vi "USB2XXXSPISlaveTest.vi"() -> ()   [LabVIEW 2010]
panel:
  out "Read Data(Hex)":string
  in  "Write Data(Hex)":string="11 22 33 44 55 66 77 88"
  in  "pConfig":T1
  in  "Channel Index":i32(ring) items=["SPI1_CS0", "SPI2_CS0"]
  in  "Device Index":i32(ring) items=["0", "1", "2", "3", "4", "5"]
  in  "Read":bool
  in  "Write":bool
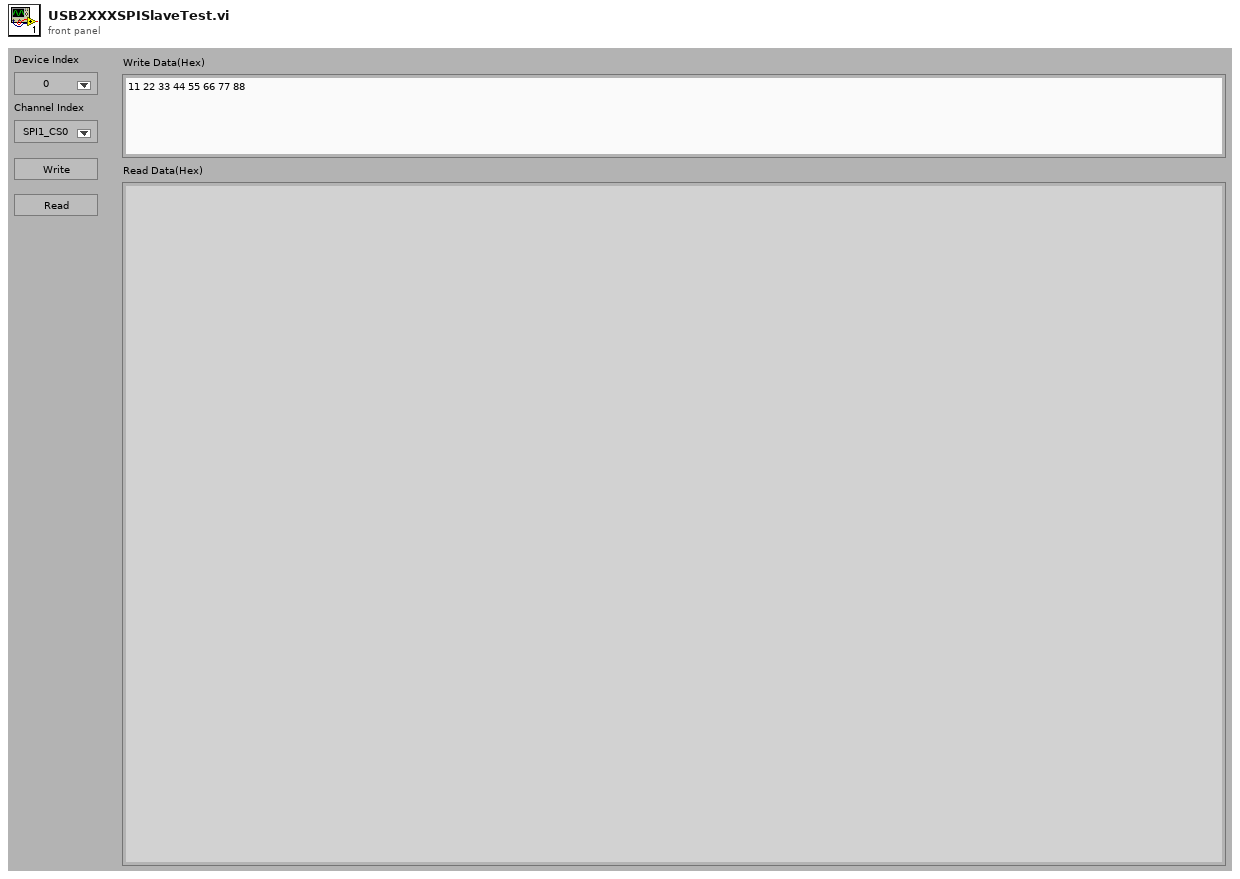
[diagram p1: front panel]
types:
  T1 = cluster{"Mode":i8, "Master":i8, "CPOL":i8, "CPHA":i8, "LSBFirst":i8, "SelPolarity":i8, "@dummy control@":i8, "@dummy control@":i8, "ClockSpeedHz":u32}
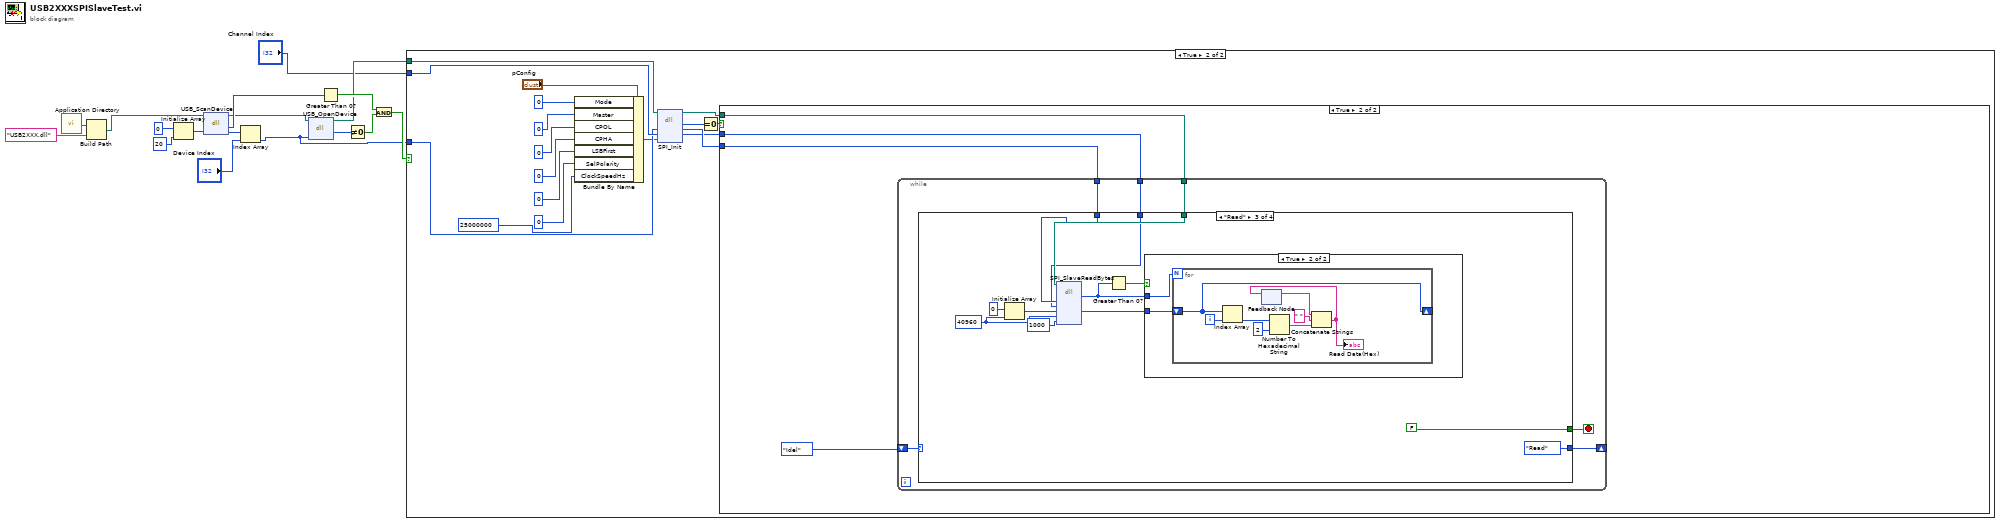
[diagram p0: block diagram]
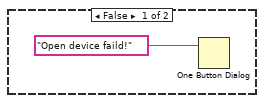
[diagram p2: hidden frame]
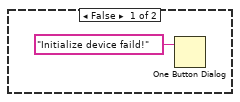
[diagram p3: hidden frame]
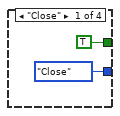
[diagram p4: hidden frame]
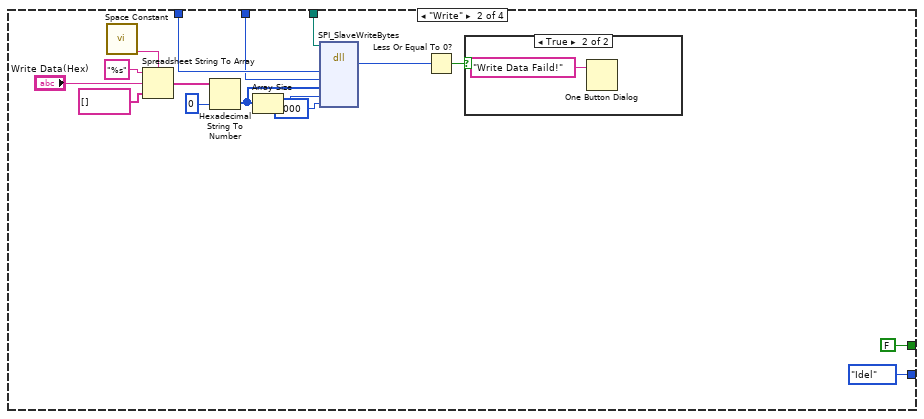
[diagram p5: hidden frame]
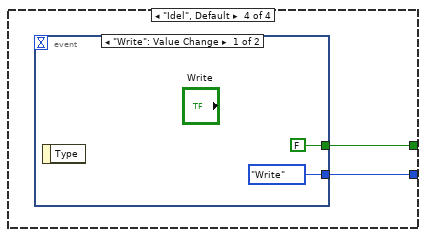
[diagram p8: hidden frame]
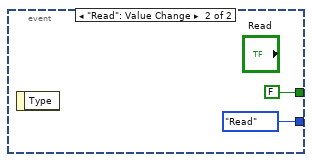
[diagram p9: hidden frame]
diagram:
  n1 = call <vilib>:"Application Directory.vi"() -> ("Application Directory"=w16:path)
  n2 = Build Path(base path=w16, name or relative path="USB2XXX.dll") -> (appended path=w10:path)
  n3 = Initialize Array(0, 20 ("dimension size")) -> (w11:i32[])
  n4 = dll-call lib="E:/Projects/USB2XXX_Example/examples/Labview/USB2SPI/USB2XXX.*" fn="USB_ScanDevice"(path in=w10, "pDevNum"=w11) -> (path out=w8:path, "return type"=w9:i32, "pDevNum"=w13:i32[])  [unwired: 2 in, 1 out]
  n5 = Index Array(array=w13, index="Device Index") -> (element=w2:i32)
  n6 = dll-call lib="E:/Projects/USB2XXX_Example/examples/Labview/USB2SPI/USB2XXX.*" fn="USB_OpenDevice"(path in=w8, "DevIndex"=w2) -> (path out=w3:path, "return type"=w7:u8)  [unwired: 3 in, 1 out]
  n7 = Greater Than 0?(x=w9) -> (x > 0?=w5:bool)
  n8 = Not Equal To 0?(x=w7) -> (x != 0?=w6:bool)
  n9 = And(x=w5, y=w6) -> (x .and. y?=w4:bool)
  n10 = case shown="True" w4 {
    tunnel: "Channel Index" -> [_ w34]
    tunnel: w2 -> [_ w33]
    tunnel: w3 -> [_ w22]
    frame False {
      n11 = One Button Dialog(message="Open device faild!") -> ()  [unwired: 1 in, 1 out]
    }
    frame True {
      n12 = Bundle By Name(cluster="pConfig", "Mode"=i8 0, "Master"=i8 0, "CPOL"=i8 0, "CPHA"=i8 0, "LSBFirst"=i8 0, "SelPolarity"=i8 0, "ClockSpeedHz"=u32 25000000) -> (w32:T1)
      n13 = dll-call lib="E:/Projects/USB2XXX_Example/examples/Labview/USB2SPI/USB2XXX.*" fn="SPI_Init"(path in=w22, "DevIndex"=w33, "SPIIndex"=w34, "pConfig"=w32) -> (path out=w21:path, "return type"=w31:i32, "DevIndex"=w20:i32, "SPIIndex"=w19:i32)  [unwired: 3 in, 1 out]
      n14 = Equal To 0?(x=w31) -> (x = 0?=w35:bool)
      n15 = case shown="True" w35 {
        tunnel: w21 -> [_ w40]
        tunnel: w20 -> [_ w39]
        tunnel: w19 -> [_ w38]
        frame False {
          n16 = One Button Dialog(message="Initialize device faild!") -> ()  [unwired: 1 in, 1 out]
        }
        frame True {
          n17 = while {
            shift-right: [w45] -> _
            shift-left: enum16{"Init", "Write", "Read", "Idel", "Close"}."Idel" ("Enum") -> [w46]
            tunnel: w40 -> [w43]
            tunnel: w39 -> [w42]
            tunnel: w38 -> [w41]
            stop <- w44 stop-if-true
            n18 = case shown="\"Read\"" w46 {
              tunnel: [enum16{"Init", "Write", "Read", "Idel", "Close"}."Close" ("Enum") enum16{"Init", "Write", "Read", "Idel", "Close"}."Idel" ("Enum") enum16{"Init", "Write", "Read", "Idel", "Close"}."Read" ("Enum") w89] -> w45
              tunnel: [TRUE FALSE FALSE w88] -> w44
              tunnel: w43 -> [_ w53 w76 _]
              tunnel: w42 -> [_ w52 w75 _]
              tunnel: w41 -> [_ w51 w74 _]
              frame "Close" {
              }
              frame "Write" {
                n19 = call <vilib>:"Space Constant.vi"() -> ("String"=w61:string)
                n20 = Spreadsheet String To Array(delimiter (Tab)=w61, format string="%s", spreadsheet string="Write Data(Hex)", array type (2D Dbl)=string[] []) -> (array=w58:string[])
                n21 = Hexadecimal String To Number(string=w58, default (0uL)=u8 0 ("default (0 U32)")) -> (number=w56:u8[])  [unwired: 1 in, 1 out]
                n22 = Array Size(array=w56) -> (size(s)=w55:i32)
                n23 = dll-call lib="E:/Projects/USB2XXX_Example/examples/Labview/USB2SPI/USB2XXX.*" fn="SPI_SlaveWriteBytes"(path in=w53, "DevHandle"=w52, "SPIIndex"=w51, "pWriteData"=w56, "WriteLen"=w55, "TimeOutMs"=1000) -> ("return type"=w50:i32)  [unwired: 7 in, 2 out]
                n24 = Less Or Equal To 0?(x=w50) -> (x <= 0?=w49:bool)
                n25 = case shown="True" w49 {
                  frame False {
                  }
                  frame True {
                    n26 = One Button Dialog(message="Write Data Faild!") -> ()  [unwired: 1 in, 1 out]
                  }
                }
              }
              frame "Read" {
                w70 = 40960 ("element")
                n27 = Initialize Array(u8 0 ("element"), w70) -> (w69:u8[])
                n28 = dll-call lib="E:/Projects/USB2XXX_Example/examples/Labview/USB2SPI/USB2XXX.*" fn="SPI_SlaveReadBytes"(path in=w76, "DevHandle"=w75, "SPIIndex"=w74, "pReadData"=w69, "ReadLen"=w70, "TimeOutMs"=1000) -> ("return type"=w67:i32, "pReadData"=w68:u8[])  [unwired: 6 in, 2 out]
                n29 = Greater Than 0?(x=w67) -> (x > 0?=w72:bool)
                n30 = case shown="True" w72 {
                  tunnel: w67 -> [_ w79]
                  tunnel: w68 -> [_ w78]
                  frame False {
                  }
                  frame True {
                    n31 = for {
                      N: w79 -> [_]
                      shift-right: [w80] -> _
                      shift-left: w78 -> [w80]
                      i -> [w87]
                      n32 = Index Array(array=w80, index=w87) -> (element=w86:u8)
                      n33 = feedback #1() -> (w84:string)  [unwired: 1 in]
                      n34 = Number To Hexadecimal String(1:i16 2 ("width (-)"), 2:w86) -> (0:w82:string)
                      n35 = Concatenate Strings(w84, " " ("string"), w82) -> (w81:string)
                      "Read Data(Hex)" <- w81
                      n36 = feedback-in #1(w81) -> ()
                    }
                  }
                }
              }
              frame "Idel", Default {
                n37 = event shown="[0] \"Write\": Value Change" {
                  selector: _ -> [_ _]
                  dyn-events: _ -> [_ _]
                  timeout: _ -> [_ _]
                  tunnel: [FALSE FALSE] -> w88
                  tunnel: [enum16{"Init", "Write", "Read", "Idel", "Close"}."Write" ("Enum") enum16{"Init", "Write", "Read", "Idel", "Close"}."Read" ("Enum")] -> w89
                  event "Write": Value Change {
                    n38 = event-data() -> ()  [unwired: 1 in, 1 out]
                  }
                  event "Read": Value Change {
                    n39 = event-data() -> ()  [unwired: 1 in, 1 out]
                  }
                }
              }
            }
          }
        }
      }
    }
  }
